vi "main 0.3.vi"() -> ()   [LabVIEW 2015]
uses:
  subvi/PHOIBOS/DEFINITIONS/DEF_dev_state.ctl
  subvi/PHOIBOS/DEFINITIONS/DEF_dev_type.ctl
  <vilib>/Utility/file.llb/Write Delimited Spreadsheet (I64).vi
  <vilib>/Utility/file.llb/Write Delimited Spreadsheet (DBL).vi
  subvi/Newport ESP301/Newport ESP301.lvlib
  subvi/sp_manip.llb/sp_manip_lib.lvlib
  subvi/sp_manip.llb/tcp_gateway.lvlib
panel:
  out "state":T1 items=["Off"=-1, "Standby"=0, "On"=1]
  in  "BasePath 2":path=path "Z:/PESdata"
  out "ESP_con?":bool caption="ESP301"
  out "phoib_con?":bool caption="PHOIBOS"
  out "manip_con?":bool caption="manipulator"
  out "cam_con?":bool caption="camera"
  in  "main_close":bool
  in  "Tab Control":enum32{"Live", "Measure", "Settings", "Devices"}(tab)
  out "cam_fps":dbl(slide)=8.239338102188393 caption="FPS" scale=0.1..50.0
  out "cam_burst_progress":u8(slide) scale=0.0..200.0
  in  "cam_burstnr":u32 max=1000
  in  "cam_burst":bool
  in  "ESP_delta":dbl
  in  "ESP_+ 2":bool
  in  "ESP_+":bool
  in  "ESP_go":bool
  in  "ESP_dest_t":dbl caption="Delay"
  in  "ESP_dest":dbl caption="Position"
  in  "ESP_set_t0":bool
  in  "phoib_I_6s":dbl=3200.0
  in  "phoib_I_5s":dbl=1400.0
  in  "phoib_I_4s":dbl=4.2
  in  "phoib_I_3s":dbl
  in  "phoib_I_2s":dbl=35.0
  in  "phoib_I_1s":dbl=21.9
  in  "phoib_standby":bool
  in  "phoib_set":bool
  out "phoib_I_6":dbl caption="Screen Voltage"
  out "phoib_I_5":dbl caption="Detctor Voltage"
  out "phoib_I_4":dbl caption="Work Function"
  out "phoib_I_3":dbl caption="Coil Current"
  out "phoib_I_2":dbl caption="Pass Energy"
  out "phoib_I_1":dbl caption="Kinetic Energy"
  out "CCD temp [°C]":i32=-12
  out "electronics temp [°C]":i32=30
  out "Saved Positions":string[][](table)=[["ertwertwert", "-2.299945", "-2.030214", "38.900024", "50.000762", "0.000887", "-97.998082"], ["uztgugt", "-14.999451", "-13.638894", "442.380066", "13.998380", "-1.893758", "-76.305838"], ["asdf", "-14.999451", "-13.638894", "442.380066", "13.998380", "-1.893758", "-76.305838"], ["test3", "-14.999451", "-13.638894", "441.380066", "13.998380", "-1.893758", "-76.305838"]]
  in  "Save Pos":bool
  in  "Load":bool
  in  "Delete":bool
  in  "ManipRel":dbl=1.0
  in  "ManipRel +":bool
  in  "ManipRel -":bool
  in  "manip.rel.select":enum32{"x", "y", "z", "polar", "tilt", "azimut"}(radio)=enum."polar"
  in  "Move Abs":bool
  in  "stop manip":bool
  in  "dest":dbl[](array[numeric])=[0.007141549166819264, -0.009888298846365134, 431.30615234375, 89.00040512814502, 1.109125024699864, -227.9162918846475] caption="destinations" format="%#.5g"
  out "names":string[](array[string])=["x", "y", "z", "polar", "tilt", "azimut"]
  out "pos":dbl[](array[numeric])=[0.007141549166819264, -0.009888298846365134, 431.30615234375, 89.00040512814502, 1.109125024699864, -227.9162918846475] caption="positions" format="%.5f"
  out "Intensity Graph":u16[][](graph)
  in  "Exposure [ms]":u32=20
  in  "Mode":T2(ring)=enum."WideAngleMode"
  in  "VoltageRange":enum16{"3.5kV", "1.5kV", "400V", "100V", "10V"}(ring)=enum."400V"
  out "ESP_pos":dbl caption="Position"
  out "ESP_delay":dbl caption="Delay"
  in  "ESP_t0":dbl caption="Time Zero @"
  in  "binning":u16(ring)=2 items=["X 1", "X 2", "X 4", "X 8"]
  in  "Gain":bool
  out "max value":u16=55
  out "phoib_I_7":dbl caption="Conversion Voltage"
  in  "phoib_I_7s":dbl
  in  "phoib_I_8s":dbl
  in  "phoib_I_9s":dbl
  out "phoib_I_8":dbl caption="FD1"
  out "phoib_I_9":dbl caption="FD2"
  out "opti_frames":dbl=25.0 caption="#steps_opti"
  out "opti_current_frame":i32=25
  out "Measurement Progress":u8(slide) scale=0.0..100.0
  out "Camera Aquisition":u8(slide) scale=0.0..100.0
  in  "Optimize":bool
  in  "OptiStepSize":dbl=-1.0 caption="Step Size"
  in  "OptiRange":dbl=25.0 caption="Range"
  in  "meas_axis":string(combo)="tilt" caption="Axis"
  in  "meas_avg":i32=60 caption="Frames2Average"
  in  "OptiCancel":bool
  out "#steps_opti":dbl=25.0
  out "current_step_opti":i32=25
  out "ETA":string
  in  "BasePath":path=path "Z:/PESdata"
  in  "Path":path=path "Z:/software/ManipulatorControl/save.txt"
  in  "ROI Bottom":i32=32
  in  "ROI Top":i32=1
  in  "ROI Right":i32=40
  in  "ROI Left":i32=1
  in  "ESP Axis":i32=1 min=1 max=3
  in  "manip_init":bool
  in  "manip_release":bool
  in  "phoib_init":bool
  in  "phoib_release":bool
  in  "ESP_init":bool
  in  "ESP_release":bool
  in  "ESP301 VISA":refnum<visa-resource-name>="COM8"
  in  "cam_boardnr":i32
  in  "cam_init":bool
  in  "cam_release":bool
  out "error out":errorcluster
  out "error out 2":errorcluster
  # "step _ of _"
  # "step _ of _"
  # "manip"
  # "phoib"
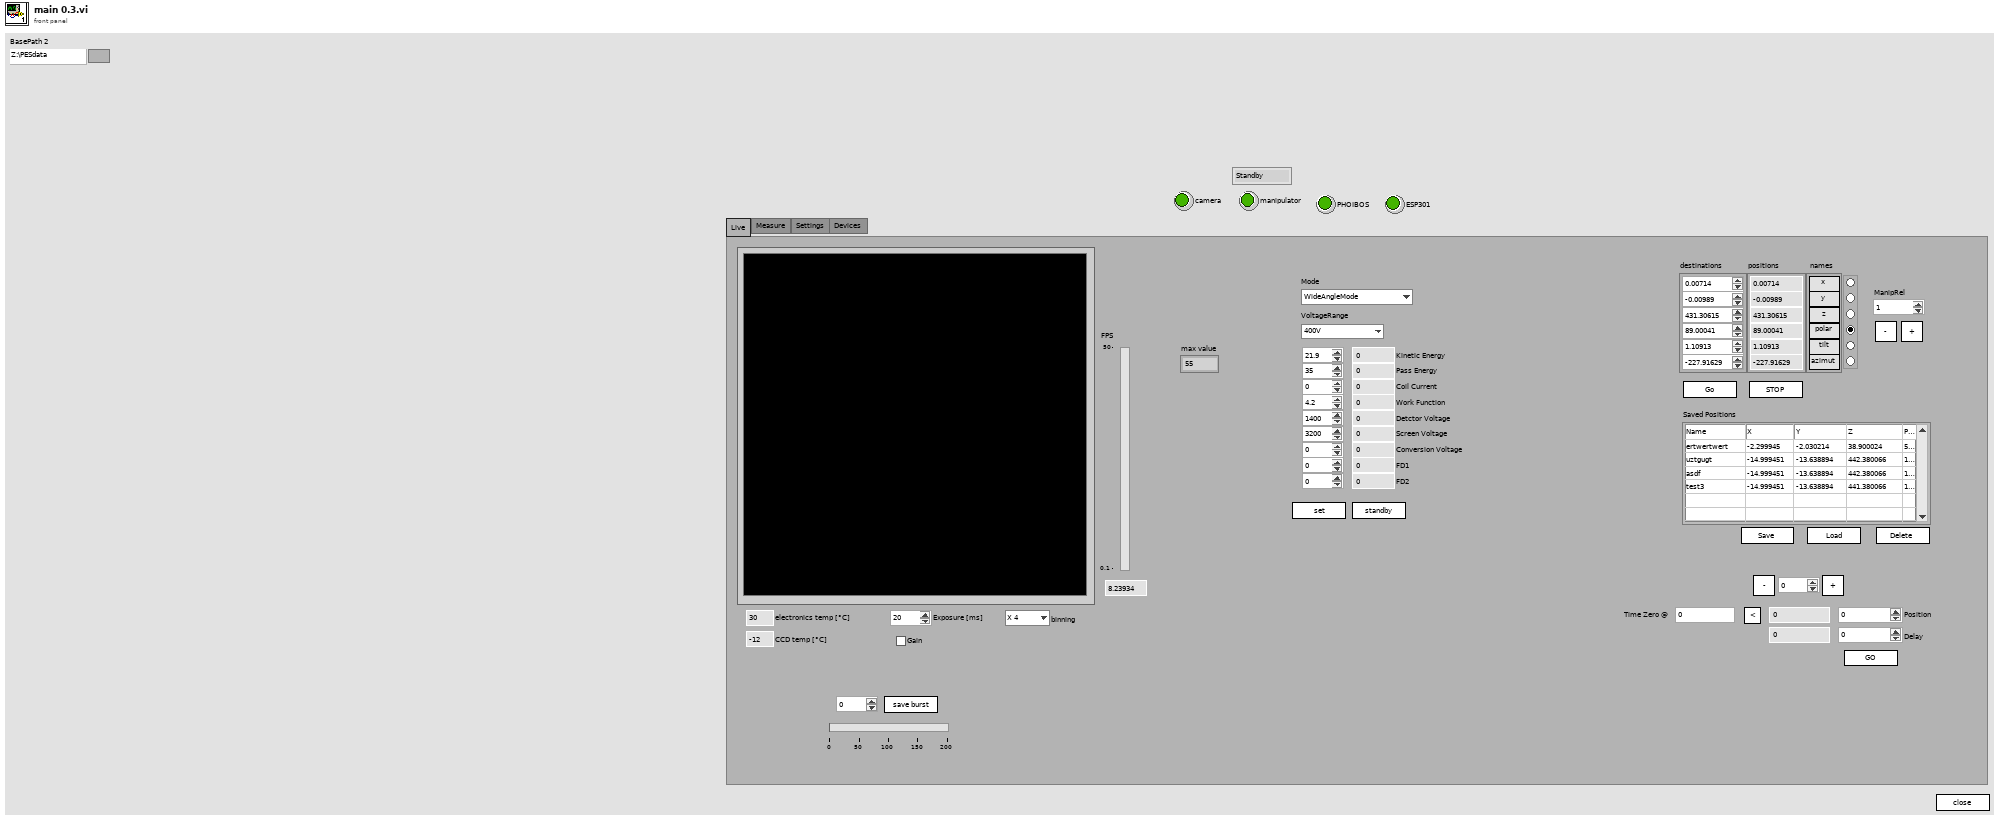
[diagram p1: front panel]
types:
  T1 = typedef "DEF_dev_state.ctl" = i32
  T2 = enum16{"HighMagnification", "MediumMagnification", "LowMagnification", "HighAngularDispersion", "MediumAngularDispersion", "LowAngularDispersion", "WideAngleMode", "LargeArea", "MediumArea", "SmallArea", "HighMagnification2", "SmallArea2", "ImagingMode"}
  T3 = cluster{"Camera type":u32, "Operating mode\nHP & QE / HS & DiCam Pro ":u32, "Frame trigger \n(High Performance and QE only)":u16, "Sequence trigger":u16, "Low Light\n(QE only)":bool, "Gain":bool, "Horzontal\nbinning":u16, "Vertical\nbinning ":u16, "ROI Left":i32, "ROI Right":i32, "ROI Top":i32, "ROI Bottom":i32}
  T4 = enum16{"open", "replace", "create", "open or create", "replace or create", "replace or create with confirmation"}
  T5 = cluster{"Axis_Name":string, "Axis_Type":string, "Axis_Position":dbl, "continous":bool, "moving":bool}[]
  T6 = cluster{"Axis_Name":string, "Axis_Type":string, "Axis_Position":dbl, "continous":bool, "moving":bool}
  T7 = typedef "DEF_dev_type.ctl" = enum32{"devA (analyzer)", "devD (detector)"}
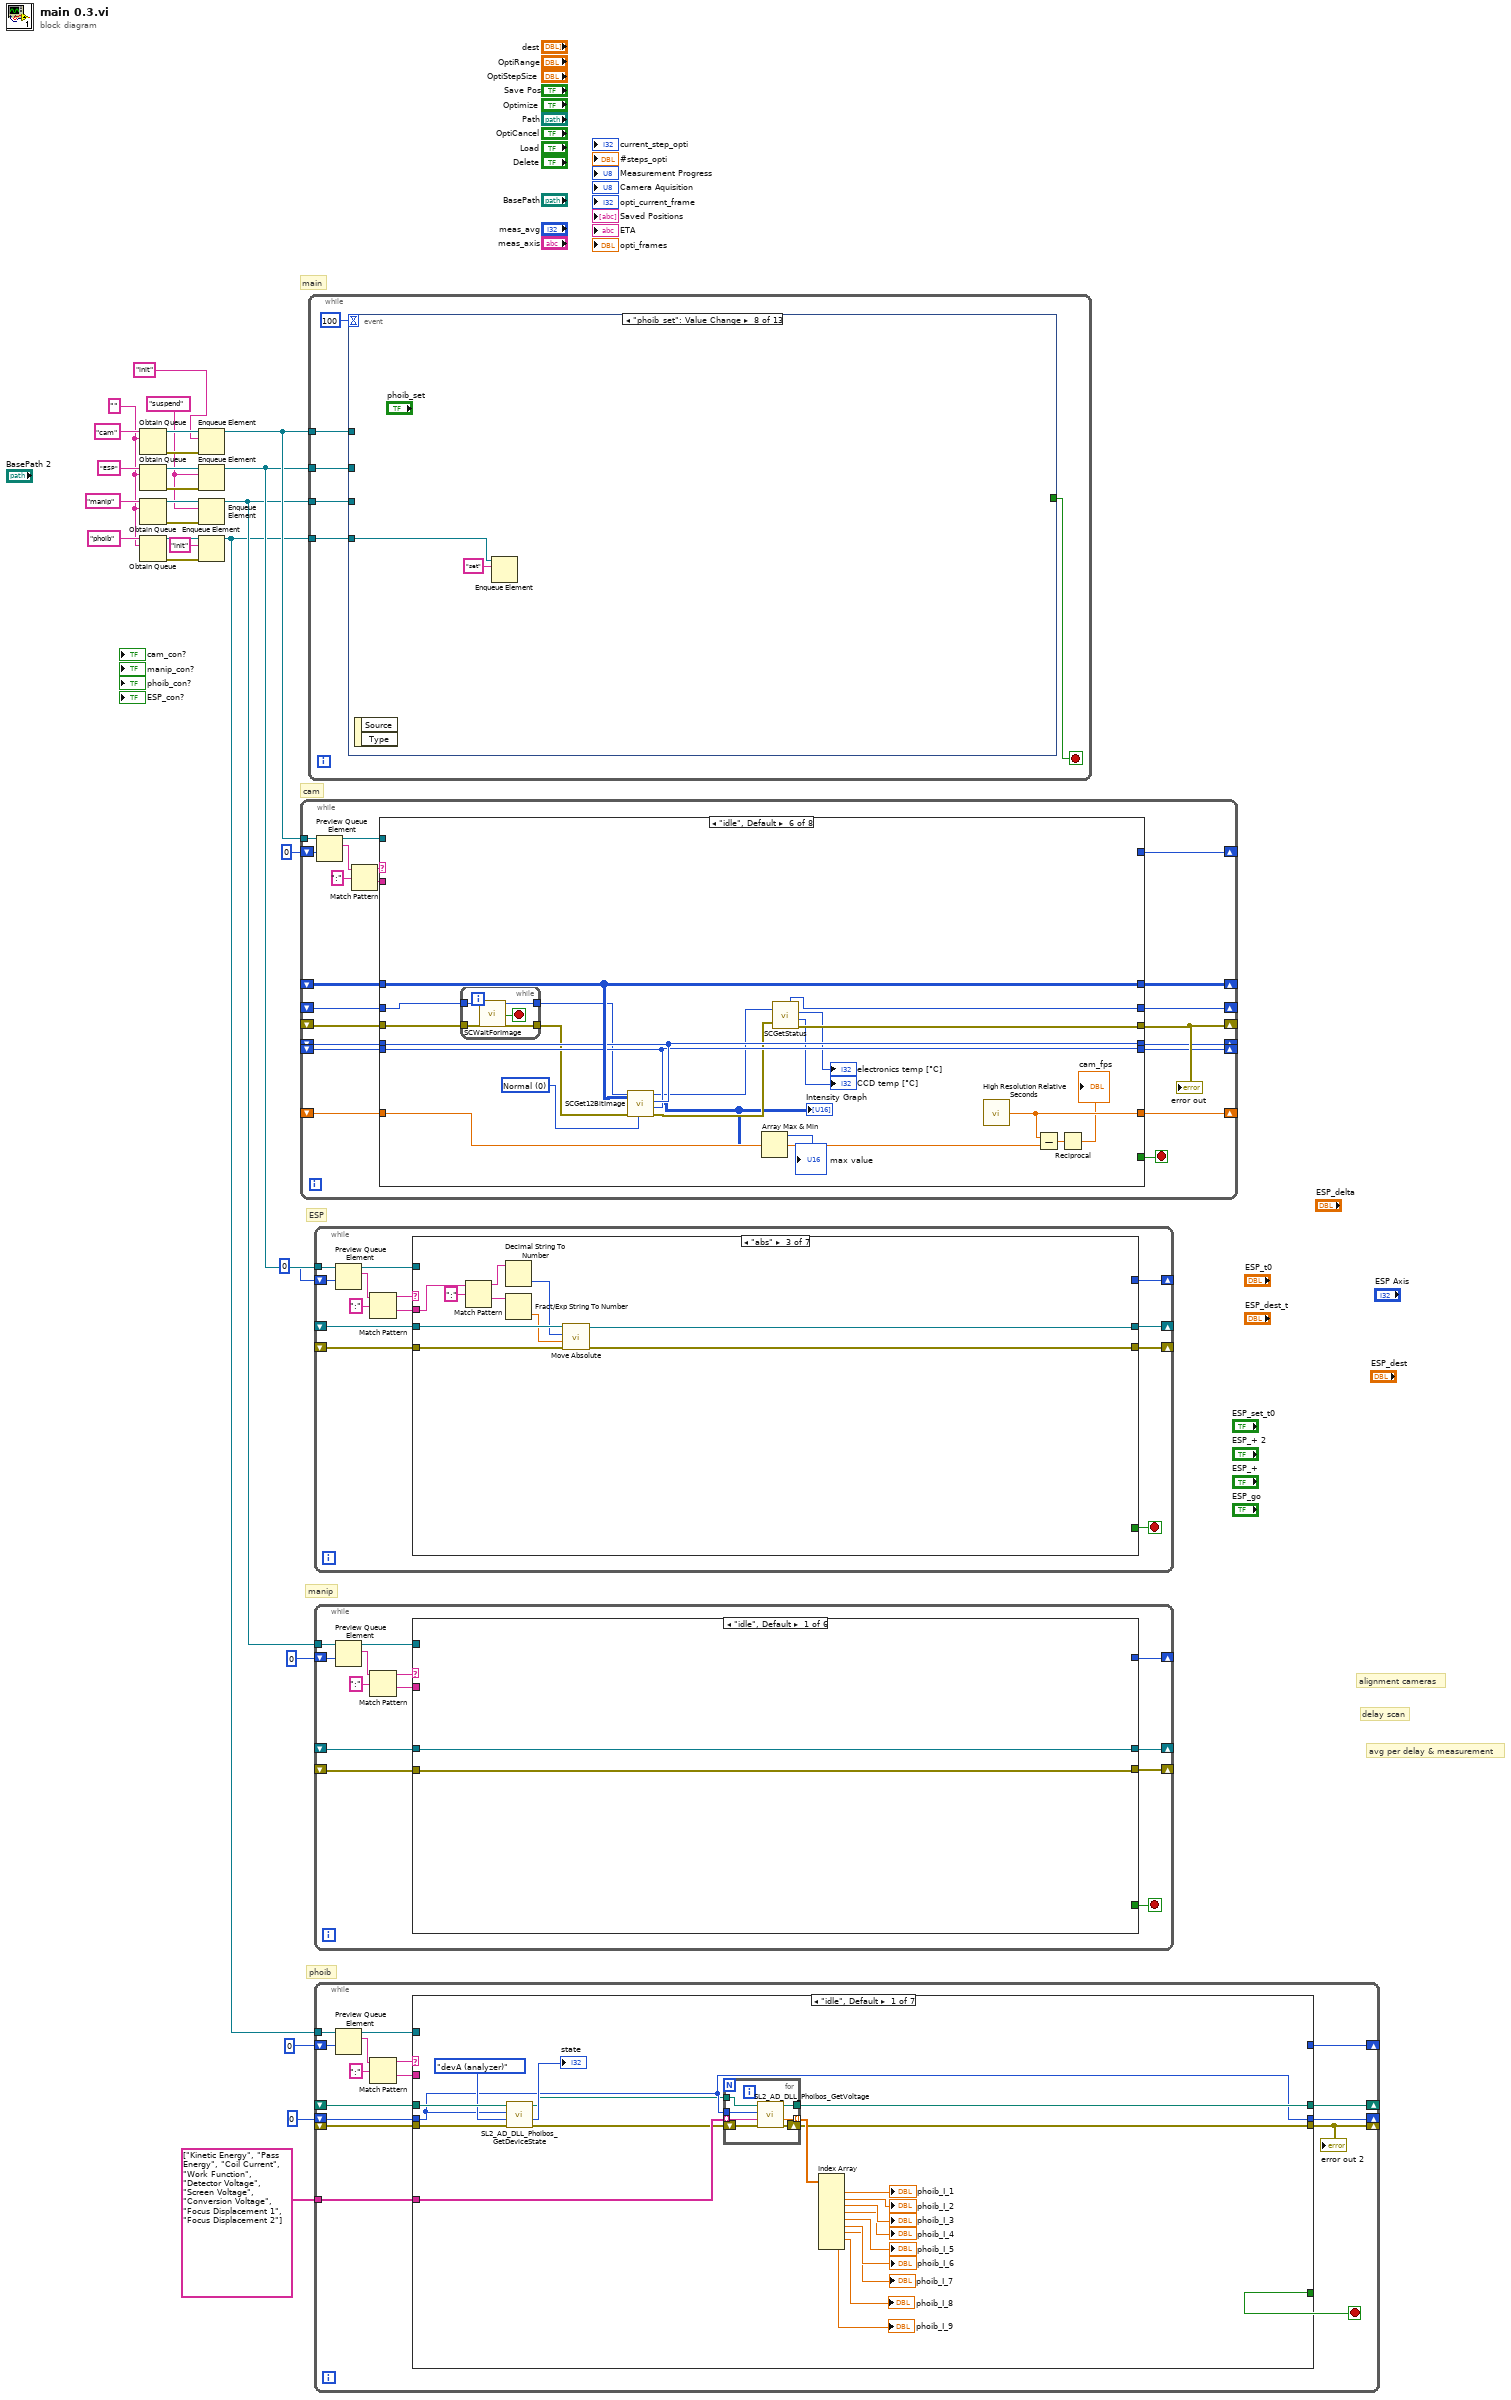
[diagram p0: block diagram]
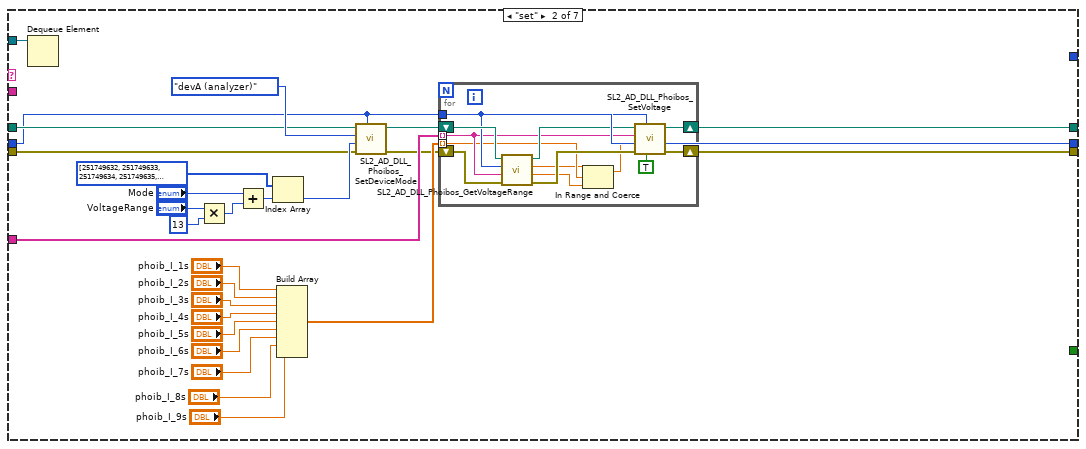
[diagram p2: hidden frame]
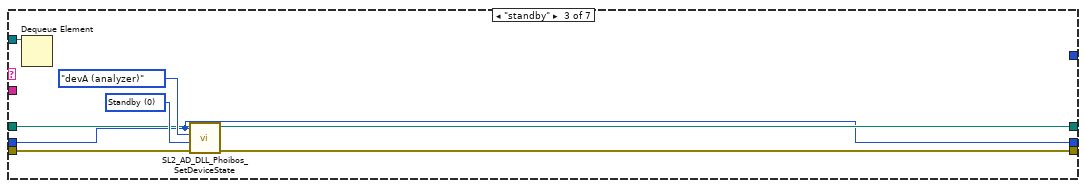
[diagram p3: hidden frame]
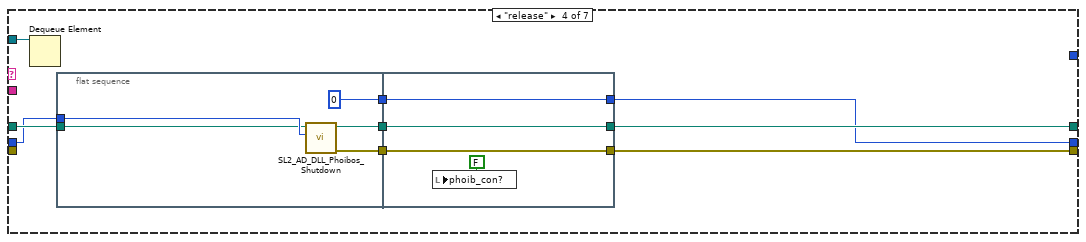
[diagram p4: hidden frame]
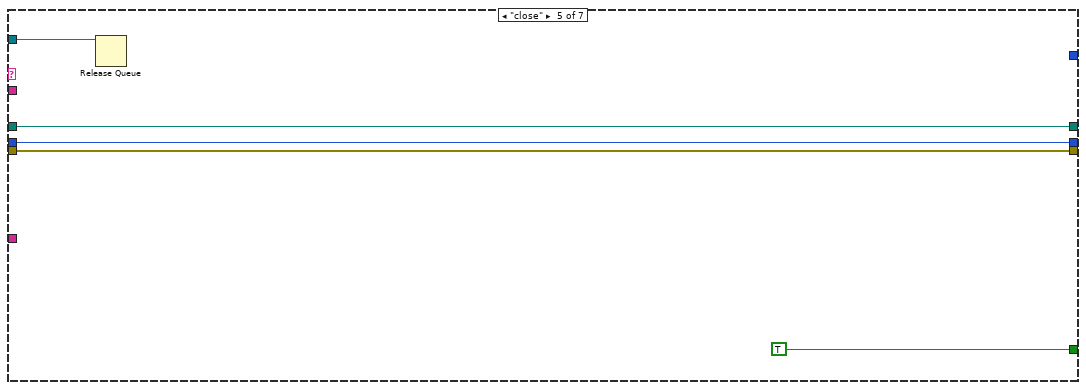
[diagram p5: hidden frame]
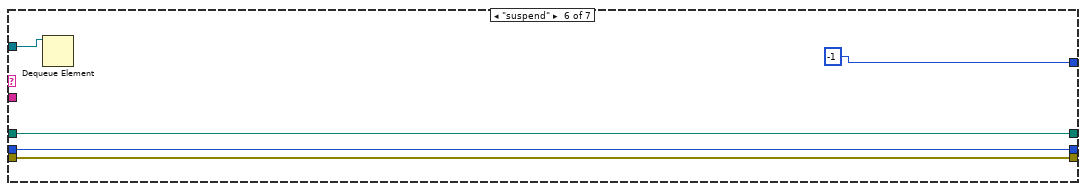
[diagram p6: hidden frame]
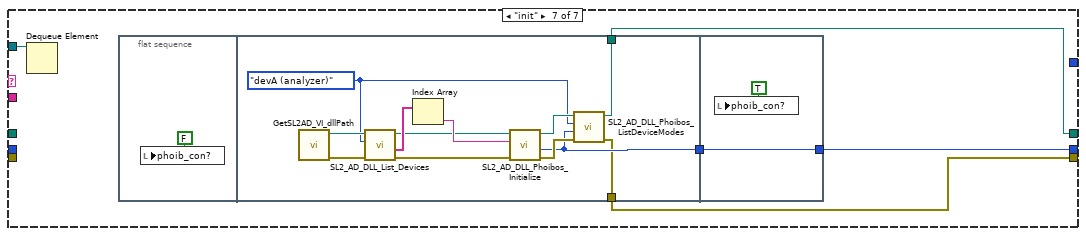
[diagram p7: hidden frame]
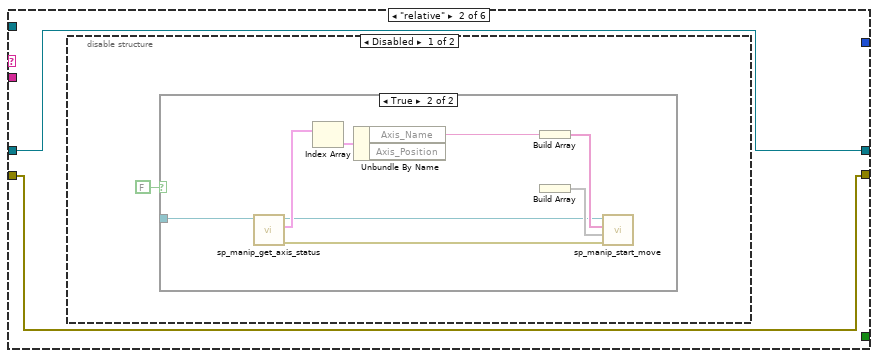
[diagram p8: hidden frame]
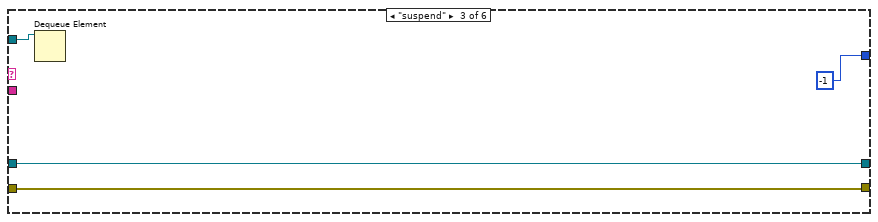
[diagram p11: hidden frame]
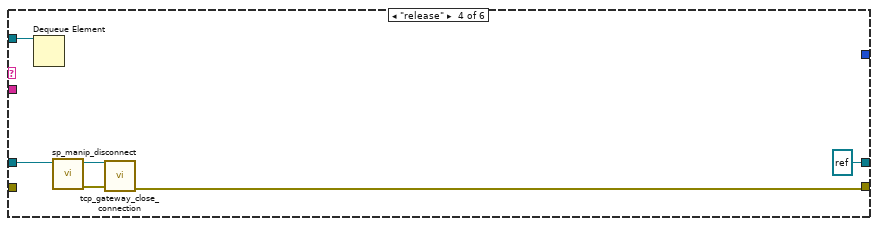
[diagram p12: hidden frame]
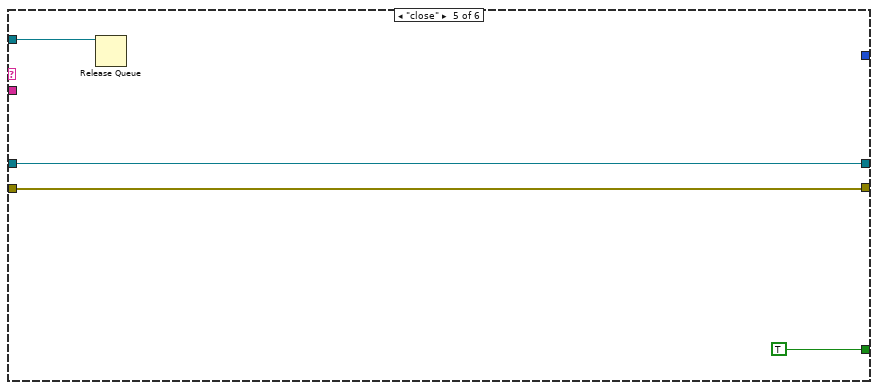
[diagram p13: hidden frame]
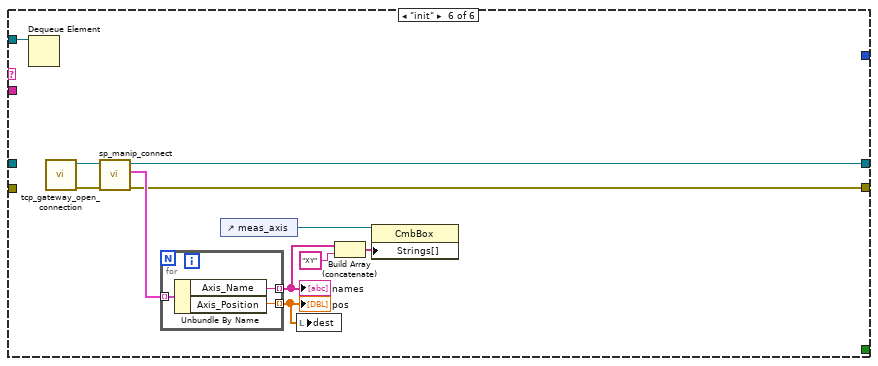
[diagram p14: hidden frame]
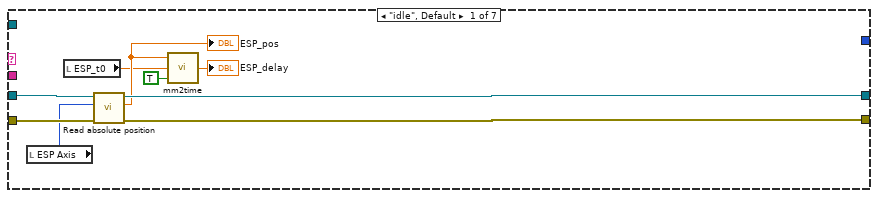
[diagram p15: hidden frame]
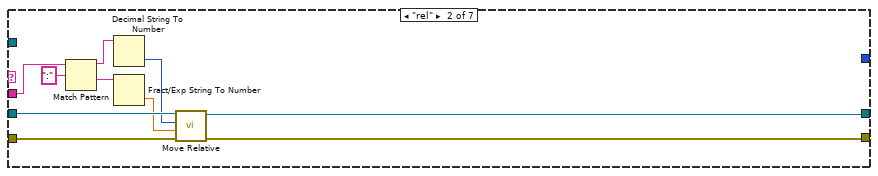
[diagram p16: hidden frame]
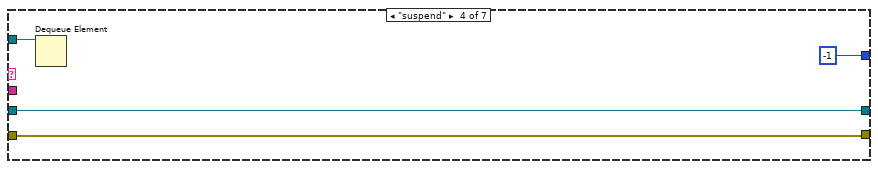
[diagram p17: hidden frame]
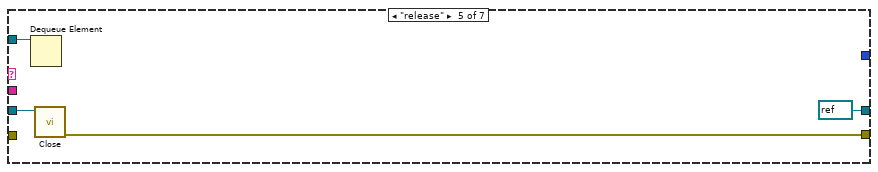
[diagram p18: hidden frame]
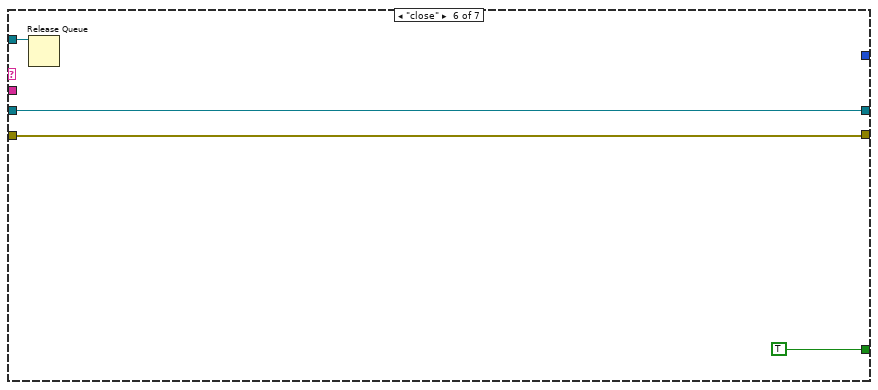
[diagram p19: hidden frame]
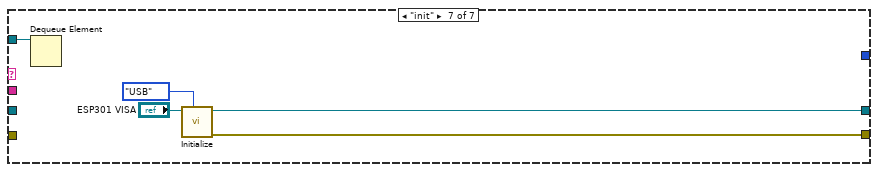
[diagram p20: hidden frame]
diagram:
  w13 = "suspend" ("name (unnamed)")
  w12 = "" ("name (unnamed)")
  # "avg per delay & measurement"
  # "delay scan"
  # "alignment cameras"
  # "phoib"
  # "manip"
  # "ESP"
  # "cam"
  # "main"
  n1 = Obtain Queue(name (unnamed)="cam", element data type=w12) -> (queue out=w25:refnum<queue>, error out=w24:errorcluster)  [unwired: 3 in, 1 out]
  n2 = Obtain Queue(name (unnamed)="ESP", element data type=w12) -> (queue out=w21:refnum<queue>, error out=w22:errorcluster)  [unwired: 3 in, 1 out]
  n3 = Obtain Queue(name (unnamed)="manip", element data type=w12) -> (queue out=w18:refnum<queue>, error out=w17:errorcluster)  [unwired: 3 in, 1 out]
  n4 = Obtain Queue(name (unnamed)="phoib", element data type=w12) -> (queue out=w15:refnum<queue>, error out=w16:errorcluster)  [unwired: 3 in, 1 out]
  n5 = Enqueue Element(queue=w25, element="init" ("name (unnamed)"), error in (no error)=w24) -> (queue out=w23:refnum<queue>)  [unwired: 1 in, 2 out]
  n6 = Enqueue Element(queue=w21, element=w13, error in (no error)=w22) -> (queue out=w11:refnum<queue>)  [unwired: 1 in, 2 out]
  n7 = Enqueue Element(queue=w18, element=w13, error in (no error)=w17) -> (queue out=w10:refnum<queue>)  [unwired: 1 in, 2 out]
  n8 = Enqueue Element(queue=w15, element="init", error in (no error)=w16) -> (queue out=w9:refnum<queue>)  [unwired: 1 in, 2 out]
  n9 = while {
    tunnel: w23 -> [w47]
    shift-right: [w41] -> _
    shift-left: _ -> [w40]
    shift-right: [w39] -> _
    shift-left: _ -> [w35]
    shift-right: [w38] -> _
    shift-left: _ -> [w34]
    shift-right: [w37] -> _
    shift-left: _ -> [w33]
    shift-right: [w36] -> _
    shift-left: _ -> [w32]
    shift-right: [w29] -> _
    shift-left: 0 -> [w30]
    shift-right: [w28] -> _
    shift-left: _ -> [w27]
    stop <- w31 stop-if-true
    n10 = Preview Queue Element(queue=w47, timeout in ms (-1)=w30) -> (queue out=w46:refnum<queue>, element=w45:string)  [unwired: 1 in, 2 out]
    n11 = Match Pattern(string=w45, regular expression=":") -> (before substring=w42:string, after substring=w43:string)  [unwired: 1 in, 2 out]
    n12 = case shown="\"idle\", Default" w42 {
      tunnel: w46 -> [w56 w80 w123 w168 w179 _ _ w235]
      tunnel: w43 -> [_ _ w136 _ _ _ w211 _]
      tunnel: [u16[][] [] w81 w133 w167 w177 w199 w209 w233] -> w41
      tunnel: w40 -> [_ _ w133 w167 w177 w199 w209 w233]
      tunnel: [w55 w82 w132 u64 0 ("Hout") w176 w190 w208 w232] -> w39
      tunnel: [w57 w83 w129 w162 w175 w193 w207 w231] -> w38
      tunnel: [0 ("Horizontal size") w73 w131 w166 w174 w198 w206 w230] -> w37
      tunnel: [0 ("Vertical size") w72 w130 w165 w173 w197 w205 w229] -> w36
      tunnel: w35 -> [_ w85 w132 w164 w176 w189 w208 w232]
      tunnel: w34 -> [_ w84 w129 _ w175 w188 w218 w231]
      tunnel: w33 -> [_ _ w131 w166 w174 w198 w206 w230]
      tunnel: w32 -> [_ _ w130 w165 w173 w197 w205 w229]
      tunnel: [_ _ _ _ TRUE _ _ _] -> w31
      tunnel: [_ _ _ _ _ _ _ -1] -> w29
      tunnel: [_ _ _ _ _ w185 _ _] -> w28
      tunnel: w27 -> [_ _ _ _ _ w184 _ _]
      frame "init" {
        n13 = Dequeue Element(queue=w56) -> (queue out=w49:refnum<queue>)  [unwired: 2 in, 3 out]
        n14 = Enqueue Element At Opposite End(queue=w49, element="set") -> ()  [unwired: 2 in, 3 out]
        n15 = flat-sequence {
          tunnel: [w59] -> w54
          tunnel: [w60] -> w53
          tunnel: [w68] -> w55
          tunnel: [w69] -> w57
          tunnel: w54 -> [w69]
          tunnel: w53 -> [w68]
          frame #0 {
            n16 = local write "cam_con?"(FALSE ("cam_con?")) -> ()
          }
          frame #1 {
            n17 = call "SCInitBoard.vi"("boardnr"="cam_boardnr") -> ("Hout"=w63:u32, "error out"=w64:errorcluster)  [unwired: 1 in, 1 out]
            n18 = call "SCSetupCamera.vi"("Handle"=w63, "error in (no error)"=w64) -> ("Hout"=w65:u64, "error out"=w66:errorcluster)  [unwired: 1 out]
            n19 = call "SCStopCOC.vi"("error in (no error)"=w66, "Stop mode"=0, "Handle"=w65) -> ("error out"=w59:errorcluster, "Hout"=w60:u64)
          }
          frame #2 {
            n20 = local write "cam_con?"(TRUE ("cam_con?")) -> ()
          }
        }
      }
      frame "set" {
        w79 = u32 1 ("Operating mode\nHP & QE / HS & DiCam Pro")
        n21 = Dequeue Element(queue=w80) -> ()  [unwired: 2 in, 4 out]
        n22 = Bundle By Name(cluster=cluster{"Delay":dbl, "Exposure ":dbl} {"Delay"=0.0, "Exposure "=0.0} ("Delay and exposure"), "Exposure"="Exposure [ms]") -> (w76:cluster{"Delay":dbl, "Exposure ":dbl})
        n23 = Bundle By Name(cluster=T3 {"Camera type"=0, "Operating mode\nHP & QE / HS & DiCam Pro "=0, "Frame trigger \n(High Performance and QE only)"=0, "Sequence trigger"=0, "Low Light\n(QE only)"=FALSE, "Gain"=FALSE, "Horzontal\nbinning"=0, "Vertical\nbinning "=0, "ROI Left"=1, "ROI Right"=20, "ROI Top"=1, "ROI Bottom"=15} ("Camera controls"), "Operating mode\nHP & QE / HS & DiCam Pro"=w79, "Horzontal\nbinning"="binning", "Vertical\nbinning"="binning", "ROI Left"="ROI Left", "ROI Right"="ROI Right", "ROI Top"="ROI Top", "ROI Bottom"="ROI Bottom", "Gain"="Gain") -> (w96:T3)
        n24 = call "New delay and exposure forma.vi"("Operating mode\nHP & QE / HS & DiCam Pro"=w79, "Delay and exposure"=w76) -> ("Output table"=w97:string)  [unwired: 3 in]
        n25 = call "SCStopCOC.vi"("error in (no error)"=w84, "Stop mode"=0, "Handle"=w85) -> ("error out"=w101:errorcluster, "Hout"=w100:u64)
        n26 = call "SCSetCoC.vi"("error in (no error)"=w101, "Delay and exposure table"=w97, "Camera controls"=w96, "Handle"=w100) -> ("error out"=w89:errorcluster, "Hout"=w88:u64)  [unwired: 1 out]
        n27 = call "SCGetImageSize.vi"("Handle"=w88, "error in (no error)"=w89) -> ("Hout"=w87:u64, "error out"=w86:errorcluster, "Horizontal size"=w73:i32, "Vertical size"=w72:i32)  [unwired: 2 out]
        n28 = Greater?(x=w73, y=w72) -> (0:w74:bool)
        n29 = Select(t=w73, s=w74, f=w72) -> (s? t:f=w71:i32)
        n30 = Initialize Array(u16 0 ("dimension size"), w72, w73) -> (w81:u16[][])
        n31 = call "SCRun.vi"("error in (no error)"=w86, "Run mode"=0, "Handle"=w87) -> ("error out"=w83:errorcluster, "Hout"=w82:u64)  [unwired: 1 out]
        n32 = property on="Intensity Graph" class="IntGraph (strict)"("XScale.Maximum"=w71, "YScale.Maximum"=w71) -> ()  [unwired: 2 in, 2 out]
      }
      frame "burst" {
        w103 = "\r"
        w104 = "\t"
        n33 = local read "Exposure [ms]"() -> (w112:u32)
        n34 = local read "binning"() -> (w114:u16)
        n35 = Dequeue Element(queue=w123) -> ()  [unwired: 2 in, 4 out]
        n36 = local read "Gain"() -> (w113:bool)
        n37 = Boolean To (0,1)(Boolean=w113) -> (0, 1=w115:i16)
        n38 = Get Date/Time In Seconds() -> (seconds since 1Jan1904=w128:timestamp)
        n39 = Match Pattern(string=w136, regular expression=":") -> (before substring=w135:string, after substring=w134:string)  [unwired: 1 in, 2 out]
        n40 = Number To Decimal String(number=w112) -> (decimal integer string=w117:string)  [unwired: 1 in]
        n41 = Number To Decimal String(number=w115) -> (decimal integer string=w119:string)  [unwired: 1 in]
        n42 = Number To Decimal String(number=w114) -> (decimal integer string=w121:string)  [unwired: 1 in]
        n43 = String To Path(string=w134) -> (path=w126:path)
        n44 = Format Date/Time String(time format string (%c)="%Y.%m.%d-%H.%M.%S", seconds (now)=w128) -> (date/time string=w125:string)  [unwired: 1 in]
        n45 = Build Path(base path=w126, name or relative path=w125) -> (appended path=w124:path)
        n46 = Decimal String To Number(string=w135) -> (number=w102:i32)  [unwired: 2 in, 1 out]
        n47 = Create Folder(path (use dialog)=w124) -> (created path=w107:path)  [unwired: 2 in, 2 out]
        n48 = Concatenate Strings("Exposure:", w104, w117, w103, "Gain:", w104, w119, w103, "binning", w104, w121, w103) -> (w111:string)
        n49 = Build Path(base path=w107, name or relative path="info.txt") -> (appended path=w106:path)
        n50 = Open/Create/Replace File(file path (use dialog)=w106, operation (0:open)=T4."replace or create") -> (refnum out=w109:refnum<file>)  [unwired: 4 in, 2 out]
        n51 = Write to Text File(file (use dialog)=w109, text=w111) -> (refnum out=w110:refnum<file>)  [unwired: 2 in, 2 out]
        n52 = Close File(refnum=w110) -> ()  [unwired: 1 in, 2 out]
        n53 = for {
          N: w102 -> [_]
          tunnel: w133 -> [w154]
          tunnel: w132 -> [w151]
          tunnel: w129 -> [w150]
          tunnel: w131 -> [w153]
          tunnel: w130 -> [w152]
          tunnel: w107 -> [w145]
          tunnel: 1000 ("x") -> [w143]
          i -> [w138]
          w155 = 0 items=["Normal", "Upside down"] ("mode")
          n54 = while {
            tunnel: [w159] -> w148
            tunnel: [w158] -> w149
            tunnel: w151 -> [w157]
            tunnel: w150 -> [w156]
            stop <- w160 stop-if-true
            n55 = call "SCWaitForImage.vi"("Handle"=w157, "error in (no error)"=w156) -> ("Hout"=w158:u64, "Image Valid"=w160:bool, "error out"=w159:errorcluster)  [unwired: 15 in]
          }
          n56 = Add(x=w143, y=w138) -> (x+y=w142:i32)
          n57 = Number To Decimal String(number=w142) -> (decimal integer string=w141:string)  [unwired: 1 in]
          n58 = String Subset(string=w141, offset (0)=1) -> (substring=w139:string)  [unwired: 1 in]
          n59 = Build Path(base path=w145, name or relative path=w139) -> (appended path=w144:path)
          n60 = call "SCGet12BitImage.vi"("mode"=w155, "Input array"=w154, "error in (no error)"=w148, "Vertical size"=w152, "Horizontal size"=w153, "Handle"=w149) -> ("error out"=w146:errorcluster, "imgdata"=w147:u16[][])  [unwired: 1 in, 1 out]
          n61 = call-poly <vilib>:"Write Delimited Spreadsheet.vi"("file path (dialog if empty)"=w144, "2D data"=w147, "error in (no error)"=w146) -> ()  [unwired: 11 in, 2 out]
          n62 = local write "Intensity Graph"(w147) -> ()
          "cam_burst_progress" <- w138
        }
        n63 = property on="cam_burst_progress" class="Slide (strict)"("Scale.Maximum"=w102) -> ()  [unwired: 2 in, 2 out]
      }
      frame "release" {
        n64 = Dequeue Element(queue=w168) -> ()  [unwired: 2 in, 4 out]
        n65 = flat-sequence {
          tunnel: w164 -> [w170]
          tunnel: [w169] -> w161
          tunnel: [w172] -> w162
          tunnel: w161 -> [w172]
          frame #0 {
            n66 = call "SCCloseBoard.vi"("Handle"=w170) -> ("error out"=w169:errorcluster)  [unwired: 1 in, 2 out]
          }
          frame #1 {
            n67 = local write "cam_con?"(FALSE ("cam_con?")) -> ()
          }
        }
      }
      frame "close" {
        n68 = Release Queue(queue=w179) -> ()  [unwired: 2 in, 3 out]
      }
      frame "idle", Default {
        w196 = 0 items=["Normal", "Upside down"] ("mode")
        n69 = while {
          tunnel: [w203] -> w186
          tunnel: [w202] -> w187
          tunnel: w189 -> [w201]
          tunnel: w188 -> [w200]
          stop <- w204 stop-if-true
          n70 = call "SCWaitForImage.vi"("Handle"=w201, "error in (no error)"=w200) -> ("Hout"=w202:u64, "Image Valid"=w204:bool, "error out"=w203:errorcluster)  [unwired: 15 in]
        }
        n71 = call "SCGet12BitImage.vi"("mode"=w196, "Input array"=w199, "error in (no error)"=w186, "Vertical size"=w197, "Horizontal size"=w198, "Handle"=w187) -> ("error out"=w194:errorcluster, "imgdata"=w181:u16[][], "Hout"=w195:u64)  [unwired: 1 in]
        "Intensity Graph" <- w181
        n72 = Array Max & Min(array=w181) -> (max value=→"max value":u16)  [unwired: 3 out]
        n73 = call "SCGetStatus.vi"("Handle"=w195, "error in (no error)"=w194) -> ("Hout"=w190:u64, "Electronics temperature"=→"electronics temp [°C]":i32, "CCD temperature"=→"CCD temp [°C]":i32, "error out"=w193:errorcluster)  [unwired: 2 out]
        n74 = call <vilib>:"High Resolution Relative Seconds.vi"() -> ("relative seconds"=w185:dbl)
        n75 = Subtract(x=w185, y=w184) -> (x-y=w183:dbl)
        n76 = Reciprocal(x=w183) -> (1/x=→"cam_fps":dbl)
      }
      frame "snap" {
        n77 = local read "BasePath 2"() -> (w220:path)
        n78 = local read "meas_avg"() -> (w215:i32)
        n79 = Initialize Array(u32 0 ("element"), w206, w205) -> (w217:u32[][])
        n80 = Build Path(base path=w220, name or relative path=w211) -> (appended path=w210:path)
        n81 = for {
          N: w215 -> [_]
          tunnel: w206 -> [w228]
          tunnel: w205 -> [w227]
          tunnel: w209 -> [w225]
          shift-right: [w222] -> w216
          shift-left: w217 -> [w224]
          shift-right: [w221] -> w207
          shift-left: w218 -> [w226]
          n82 = call "SCGet12BitImage.vi"("Input array"=w225, "error in (no error)"=w226, "Vertical size"=w227, "Horizontal size"=w228) -> ("error out"=w221:errorcluster, "imgdata"=w223:u16[][])  [unwired: 3 in, 1 out]
          n83 = Add(x=w223, y=w224) -> (x+y=w222:u32[][])
        }
        n84 = Divide(x=w216, y=w215) -> (x/y=w214:dbl[][])
        n85 = call-poly <vilib>:"Write Delimited Spreadsheet.vi"("file path (dialog if empty)"=w210, "format (%.3f)"="%d", "2D data"=w214, "transpose? (F)"=TRUE) -> ()  [unwired: 10 in, 2 out]
      }
      frame "suspend" {
        n86 = Dequeue Element(queue=w235) -> ()  [unwired: 2 in, 4 out]
      }
    }
    "error out" <- w38
  }
  n87 = while {
    tunnel: w23 -> [w239]
    tunnel: w11 -> [w238]
    tunnel: w10 -> [w237]
    tunnel: w9 -> [w236]
    stop <- w241 stop-if-true
    n88 = event shown="[7] \"phoib_set\": Value Change" {
      selector: _ -> [_ _ _ _ _ _ _ _ _ _ _ _ _]
      dyn-events: _ -> [_ _ _ _ _ _ _ _ _ _ _ _ _]
      timeout: 100 -> [_ _ _ _ _ _ _ _ _ _ _ _ _]
      tunnel: [_ TRUE _ _ _ _ _ _ _ _ _ _ _] -> w241
      tunnel: w239 -> [_ w251 w254 _ _ _ _ _ w280 w281 _ _ _]
      tunnel: w238 -> [_ w250 _ w258 _ _ _ _ _ _ _ _ _]
      tunnel: w237 -> [_ w249 _ _ w264 _ _ _ _ _ _ _ _]
      tunnel: w236 -> [_ w248 _ _ _ w270 w276 w277 _ _ _ _ _]
      event Timeout {
        n89 = event-data() -> ()  [unwired: 1 in, 1 out]
      }
      event "main_close": Value Change {
        w242 = "close" ("element")
        w247 = "release" ("element")
        n90 = event-data() -> ()  [unwired: 1 in, 1 out]
        n91 = Enqueue Element(queue=w251, element=w247) -> (queue out=w246:refnum<queue>)  [unwired: 2 in, 2 out]
        n92 = Enqueue Element(queue=w250, element=w247) -> (queue out=w245:refnum<queue>)  [unwired: 2 in, 2 out]
        n93 = Enqueue Element(queue=w249, element=w247) -> (queue out=w244:refnum<queue>)  [unwired: 2 in, 2 out]
        n94 = Enqueue Element(queue=w248, element=w247) -> (queue out=w243:refnum<queue>)  [unwired: 2 in, 2 out]
        n95 = Enqueue Element(queue=w246, element=w242) -> ()  [unwired: 2 in, 3 out]
        n96 = Enqueue Element(queue=w245, element=w242) -> ()  [unwired: 2 in, 3 out]
        n97 = Enqueue Element(queue=w244, element=w242) -> ()  [unwired: 2 in, 3 out]
        n98 = Enqueue Element(queue=w243, element=w242) -> ()  [unwired: 2 in, 3 out]
      }
      event "cam_release", "cam_init": Value Change {
        n99 = event-data() -> ()  [unwired: 1 in, 2 out]
        n100 = Select(t="init" ("name (unnamed)"), s="cam_init", f="release" ("name (unnamed)")) -> (s? t:f=w253:string)
        n101 = Enqueue Element(queue=w254, element=w253) -> ()  [unwired: 2 in, 3 out]
      }
      event "ESP_release", "ESP_init": Value Change {
        n102 = event-data() -> ()  [unwired: 1 in, 2 out]
        n103 = Select(t="init" ("name (unnamed)"), s="ESP_init", f="release" ("name (unnamed)")) -> (s? t:f=w262:string)
        n104 = Enqueue Element(queue=w258, element=w262) -> ()  [unwired: 2 in, 3 out]
      }
      event "manip_init", "manip_release": Value Change {
        n105 = event-data() -> ()  [unwired: 1 in, 2 out]
        n106 = Flush Queue(queue=w264) -> (queue out=w263:refnum<queue>)  [unwired: 1 in, 2 out]
        n107 = Select(t="init" ("name (unnamed)"), s="manip_init", f="release" ("name (unnamed)")) -> (s? t:f=w266:string)
        n108 = Enqueue Element(queue=w263, element=w266) -> ()  [unwired: 2 in, 3 out]
      }
      event "phoib_release", "phoib_init": Value Change {
        n109 = event-data() -> ()  [unwired: 1 in, 2 out]
        n110 = Flush Queue(queue=w270) -> (queue out=w269:refnum<queue>)  [unwired: 1 in, 2 out]
        n111 = Select(t="init" ("name (unnamed)"), s="phoib_init", f="release" ("name (unnamed)")) -> (s? t:f=w272:string)
        n112 = Enqueue Element(queue=w269, element=w272) -> ()  [unwired: 2 in, 3 out]
      }
      event "phoib_standby": Value Change {
        n113 = event-data() -> ()  [unwired: 1 in, 2 out]
        n114 = Enqueue Element(queue=w276, element="standby") -> ()  [unwired: 2 in, 3 out]
      }
      event "phoib_set": Value Change {
        n115 = event-data() -> ()  [unwired: 1 in, 2 out]
        n116 = Enqueue Element(queue=w277, element="set") -> ()  [unwired: 2 in, 3 out]
      }
      event "ROI Left", "ROI Right", "ROI Top", "ROI Bottom", "Exposure [ms]", "binning", "Gain": Value Change {
        n117 = event-data() -> ()  [unwired: 1 in, 6 out]
        n118 = Enqueue Element(queue=w280, element="set") -> ()  [unwired: 2 in, 3 out]
      }
      event "cam_burst": Value Change {
        n119 = event-data() -> ()  [unwired: 1 in, 1 out]
        n120 = local read "BasePath"() -> (w285:path)
        n121 = call "File Dialog"("start path"=w285) -> ("selected path"=w283:path, "cancelled"=w284:bool, "error out"=w282:errorcluster)  [unwired: 11 in, 1 out]
        n122 = case shown="False" w284 {
          tunnel: w283 -> [w288 _]
          tunnel: w282 -> [_ _]
          tunnel: w281 -> [w293 _]
          frame False {
            n123 = Path To String(path=w288) -> (string=w287:string)
            n124 = Number To Decimal String(number="cam_burstnr") -> (decimal integer string=w290:string)  [unwired: 1 in]
            n125 = Concatenate Strings("burst:" ("string"), w290, ":" ("string"), w287) -> (w286:string)
            n126 = Enqueue Element(queue=w293, element=w286) -> ()  [unwired: 2 in, 3 out]
          }
          frame True {
          }
        }
      }
      event "Move Abs": Value Change {
        n127 = event-data() -> ()  [unwired: 1 in, 1 out]
      }
      event "ManipRel +", "ManipRel -": Value Change {
        n128 = event-data() -> ()  [unwired: 1 in, 2 out]
        n129 = Negate(x="ManipRel") -> (-x=w295:dbl)
        n130 = Select(t=w295, s="ManipRel -", f="ManipRel") -> ()  [unwired: 1 out]
      }
      event "stop manip": Value Change {
        n131 = event-data() -> ()  [unwired: 1 in, 1 out]
      }
    }
  }
  n132 = while {
    tunnel: w11 -> [w304]
    shift-right: [w302] -> _
    shift-left: _ -> [w300]
    shift-right: [w301] -> _
    shift-left: _ -> [w299]
    shift-right: [w297] -> _
    shift-left: 0 -> [w298]
    stop <- w303 stop-if-true
    n133 = Preview Queue Element(queue=w304, timeout in ms (-1)=w298) -> (queue out=w307:refnum<queue>, element=w308:string)  [unwired: 1 in, 2 out]
    n134 = Match Pattern(string=w308, regular expression=":") -> (before substring=w306:string, after substring=w305:string)  [unwired: 1 in, 2 out]
    n135 = case shown="\"abs\"" w306 {
      tunnel: w307 -> [_ _ _ w342 w343 w350 w355]
      tunnel: w305 -> [_ w323 w335 _ _ _ _]
      tunnel: [_ _ _ _ _ TRUE _] -> w303
      tunnel: [w316 w325 w331 w340 refnum<visa-resource-name> refnum ("VISA resource name out") w347 w352] -> w302
      tunnel: [w315 w326 w332 w339 w345 w348 w351] -> w301
      tunnel: w300 -> [w318 w328 w333 w340 w346 w347 _]
      tunnel: w299 -> [w317 w327 w334 w339 _ w348 _]
      tunnel: [_ _ _ -1 _ _ _] -> w297
      frame "idle", Default {
        n136 = local read "ESP Axis"() -> (w310:i32)
        n137 = local read "ESP_t0"() -> (w313:dbl)
        n138 = call "Read absolute position.vi"("error in (no error)"=w317, "Axis (1)"=w310, "VISA resource name"=w318) -> ("error out"=w315:errorcluster, "Position (units)"=w314:dbl, "VISA resource name out"=w316:refnum<visa-resource-name>)  [unwired: 2 in]
        "ESP_pos" <- w314
        n139 = call "mm2time.vi"("fs?"=TRUE, "Offset (mm)"=w313, "distance (mm)"=w314) -> ("time in fs/ps seconds"=→"ESP_delay":dbl)
      }
      frame "rel" {
        n140 = Match Pattern(string=w323, regular expression=":") -> (before substring=w322:string, after substring=w321:string)  [unwired: 1 in, 2 out]
        n141 = Decimal String To Number(string=w322) -> (number=w320:i32)  [unwired: 2 in, 1 out]
        n142 = Fract/Exp String To Number(string=w321) -> (number=w319:dbl)  [unwired: 3 in, 1 out]
        n143 = call "Move Relative.vi"("error in (no error)"=w327, "Position (0 units)"=w319, "Axis (1)"=w320, "VISA resource name"=w328) -> ("error out"=w326:errorcluster, "VISA resource name out"=w325:refnum<visa-resource-name>)  [unwired: 2 in]
      }
      frame "abs" {
        n144 = Match Pattern(string=w335, regular expression=":") -> (before substring=w337:string, after substring=w336:string)  [unwired: 1 in, 2 out]
        n145 = Decimal String To Number(string=w337) -> (number=w330:i32)  [unwired: 2 in, 1 out]
        n146 = Fract/Exp String To Number(string=w336) -> (number=w329:dbl)  [unwired: 3 in, 1 out]
        n147 = call "Move Absolute.vi"("error in (no error)"=w334, "Position (0 units)"=w329, "Axis (1)"=w330, "VISA resource name"=w333) -> ("error out"=w332:errorcluster, "VISA resource name out"=w331:refnum<visa-resource-name>)  [unwired: 2 in]
      }
      frame "suspend" {
        n148 = Dequeue Element(queue=w342) -> ()  [unwired: 2 in, 4 out]
      }
      frame "release" {
        n149 = Dequeue Element(queue=w343) -> ()  [unwired: 2 in, 4 out]
        n150 = call "Close.vi"("VISA resource name"=w346) -> ("error out"=w345:errorcluster)  [unwired: 10 in]
      }
      frame "close" {
        n151 = Release Queue(queue=w350) -> ()  [unwired: 2 in, 3 out]
      }
      frame "init" {
        n152 = Dequeue Element(queue=w355) -> ()  [unwired: 2 in, 4 out]
        n153 = call "Initialize.vi"("VISA resource name"="ESP301 VISA", "Serial Link (RS232)"=enum16{"RS232", "USB"}."USB") -> ("VISA resource name out"=w352:refnum<visa-resource-name>, "error out"=w351:errorcluster)  [unwired: 7 in]
      }
    }
  }
  n154 = while {
    tunnel: w10 -> [w363]
    shift-right: [w361] -> _
    shift-left: _ -> [w359]
    shift-right: [w360] -> _
    shift-left: _ -> [w358]
    shift-right: [w356] -> _
    shift-left: 0 -> [w357]
    stop <- w362 stop-if-true
    n155 = Preview Queue Element(queue=w363, timeout in ms (-1)=w357) -> (queue out=w366:refnum<queue>, element=w367:string)  [unwired: 1 in, 2 out]
    n156 = Match Pattern(string=w367, regular expression=":") -> (before substring=w365:string, after substring=w364:string)  [unwired: 1 in, 2 out]
    n157 = case shown="\"idle\", Default" w365 {
      tunnel: w366 -> [_ _ w384 w388 w397 w408]
      tunnel: w364 -> [_ _ _ _ _ _]
      tunnel: [_ _ _ _ TRUE _] -> w362
      tunnel: [w370 w372 w386 refnum<k5> refnum ("gateway_connection out") w395 w399] -> w361
      tunnel: [w369 w371 w385 w390 w394 w398] -> w360
      tunnel: w359 -> [w370 w372 w386 w392 w395 _]
      tunnel: w358 -> [w369 w371 w385 _ w394 _]
      tunnel: [_ _ -1 _ _ _] -> w356
      frame "idle", Default {
      }
      frame "relative" {
        n158 = disable-structure shown="Disabled" {
          frame Disabled {
            n159 = case shown="True" FALSE {
              tunnel: [_ w382] -> w374
              frame False {
              }
              frame True {
                n160 = call "sp_manip_get_axis_status.vi"("gateway_connection"=w382) -> ("error out"=w377:errorcluster, "axis_out"=w381:T5, "gateway_connection out"=w375:refnum<k5>)  [unwired: 6 in, 2 out]
                n161 = Index Array(array=w381) -> (element=w380:T6, index=w383:i32)
                n162 = Unbundle By Name(w380) -> ("Axis_Name"=w376:string)  [unwired: 1 out]
                n163 = Build Array(w376) -> (w379:string[])
                n164 = Build Array() -> (w378:void[])  [unwired: 1 in]
                n165 = call "sp_manip_start_move.vi"("error in"=w377, "target positions"=w378, "axis names"=w379, "gateway_connection"=w375) -> ()  [unwired: 4 in, 4 out]
              }
            }
          }
          frame Enabled {
          }
        }
      }
      frame "suspend" {
        n166 = Dequeue Element(queue=w384) -> ()  [unwired: 2 in, 4 out]
      }
      frame "release" {
        n167 = Dequeue Element(queue=w388) -> ()  [unwired: 2 in, 4 out]
        n168 = call "sp_manip_disconnect.vi"("gateway_connection"=w392) -> ("error out"=w391:errorcluster, "gateway_connection_out"=w393:refnum<k5>)  [unwired: 7 in, 2 out]
        n169 = call "tcp_gateway_close_connection.vi"("error in"=w391, "server_connection"=w393) -> ("error out"=w390:errorcluster)  [unwired: 5 in]
      }
      frame "close" {
        n170 = Release Queue(queue=w397) -> ()  [unwired: 2 in, 3 out]
      }
      frame "init" {
        n171 = Dequeue Element(queue=w408) -> ()  [unwired: 2 in, 4 out]
        n172 = call "tcp_gateway_open_connection.vi"() -> ("gateway_connection"=w403:refnum<k5>, "error out"=w402:errorcluster)  [unwired: 5 in, 3 out]
        n173 = call "sp_manip_connect.vi"("error in"=w402, "gateway_connection"=w403) -> ("error out"=w398:errorcluster, "axis_out"=w401:T5, "gateway_connection out"=w399:refnum<k5>)  [unwired: 5 in, 2 out]
        n174 = for {
          tunnel: w401 -> [w411] mode=indexing
          tunnel: [w410] -> w406 mode=indexing
          tunnel: [w409] -> w407 mode=indexing
          n175 = Unbundle By Name(w411) -> ("Axis_Name"=w410:string, "Axis_Position"=w409:dbl)
        }
        "names" <- w406
        "pos" <- w407
        n176 = control-ref of="meas_axis"() -> (w400:refnum<vi>)
        n177 = local write "dest"(w407) -> ()
        n178 = Build Array (concatenate)(w406, "XY") -> (w404:string[])
        n179 = property on="Property Node" class="CmbBox"(reference=w400, "Strings[]"=w404) -> ()  [unwired: 1 in, 2 out]
      }
    }
  }
  n180 = while {
    tunnel: w9 -> [w422]
    shift-right: [w419] -> _
    shift-left: 0 -> [w420]
    shift-right: [w418] -> _
    shift-left: _ -> [w417]
    shift-right: [w416] -> _
    shift-left: _ -> [w415]
    shift-right: [w414] -> _
    shift-left: u32 0 ("pHandle") -> [w413]
    tunnel: string[] ["Kinetic Energy", "Pass Energy", "Coil Current", "Work Function", "Detector Voltage", "Screen Voltage", "Conversion Voltage", "Focus Displacement 1", "Focus Displacement 2"] -> [w412]
    stop <- w421 stop-if-true
    n181 = Preview Queue Element(queue=w422, timeout in ms (-1)=w420) -> (queue out=w425:refnum<queue>, element=w426:string)  [unwired: 1 in, 2 out]
    n182 = Match Pattern(string=w426, regular expression=":") -> (before substring=w424:string, after substring=w423:string)  [unwired: 1 in, 2 out]
    n183 = case shown="\"idle\", Default" w424 {
      tunnel: w425 -> [_ w479 w495 w511 w525 w529 w535]
      tunnel: w423 -> [_ _ _ _ _ _ _]
      tunnel: [_ _ _ _ TRUE _ _] -> w421
      tunnel: [_ _ _ _ _ -1 _] -> w419
      tunnel: [w436 w481 w498 w509 w523 w528 w532] -> w418
      tunnel: w417 -> [w447 w470 w500 w510 w523 w528 _]
      tunnel: [w435 w480 w497 w508 w521 w526 w531] -> w416
      tunnel: w415 -> [w445 w469 w499 _ w521 w526 _]
      tunnel: [w433 w467 w496 w507 w522 w527 w534] -> w414
      tunnel: w413 -> [w433 w467 w496 w506 w522 w527 _]
      tunnel: w412 -> [w434 w460 _ _ _ _ _]
      frame "idle", Default {
        n184 = call "SL2_AD_DLL_Phoibos_GetDeviceState.vi"("dll_path"=w447, "pHandle_in"=w433, "dev_type"=DEF_dev_type."devA (analyzer)", "error in"=w445) -> ("path out"=w432:path, "state"=→"state":T1, "error out"=w431:errorcluster)  [unwired: 2 in]
        n185 = for {
          tunnel: w433 -> [w454]
          tunnel: w434 -> [w452] mode=indexing
          tunnel: [w451] -> w444 mode=indexing
          tunnel: [w450] -> w436
          shift-right: [w449] -> w435
          shift-left: w431 -> [w453]
          tunnel: w432 -> [w448]
          n186 = call "SL2_AD_DLL_Phoibos_GetVoltage.vi"("error in"=w453, "voltage_name"=w452, "pHandle"=w454, "dll path in"=w448) -> ("error out"=w449:errorcluster, "value"=w451:dbl, "dll path out"=w450:path)  [unwired: 3 in]
        }
        n187 = Index Array(array=w444) -> (element #1=→"phoib_I_1":dbl, element #2=→"phoib_I_2":dbl, element #3=→"phoib_I_3":dbl, element #4=→"phoib_I_4":dbl, element #5=→"phoib_I_5":dbl, element #6=→"phoib_I_6":dbl, element #7=→"phoib_I_7":dbl, element #8=→"phoib_I_8":dbl, element #9=→"phoib_I_9":dbl)  [unwired: 9 in]
      }
      frame "set" {
        n188 = Dequeue Element(queue=w479) -> ()  [unwired: 2 in, 4 out]
        n189 = Multiply(x="VoltageRange", y=13) -> (x*y=w476:i32)
        n190 = Add(x="Mode", y=w476) -> (x+y=w473:i32)
        n191 = Index Array(array=u32[] [251749632, 251749633, 251749634, 251749635, 251749636, 251749637, 251749638, 251749639, 251749640, 251749641, 251749642, 251749643, 251749644, 251749645, 251749646, 251749647, 251749648, 251749649, 251749650, 251749651, 251749652, 251749653, 251749654, 251749655, 251749656, 251749657, 251749658, 251749659, 251749660, 251749661, 251749662, 251749663, 251749664, 251749665, 251749666, 251749667, 251749668, 251749669, 251749670, 251749671, 251749672, 251749673, 251749674, 251749675, 251749676, 251749677, 251749678, 251749679, 251749680, 251749681, 251749682, 251749683, 251749684, 251749685, 251749686, 251749687, 251749688, 251749689, 251749690, 251749691, 251749692, 251749693, 251749694, 251749695, 251749696] ("modeIDs"), index=w473) -> (element=w471:u32)
        n192 = Build Array("phoib_I_1s", "phoib_I_2s", "phoib_I_3s", "phoib_I_4s", "phoib_I_5s", "phoib_I_6s", "phoib_I_7s", "phoib_I_8s", "phoib_I_9s") -> (w459:dbl[])
        n193 = call "SL2_AD_DLL_Phoibos_SetDeviceMode.vi"("pHandle"=w467, "error in"=w469, "value"=w471, "dev_type"=DEF_dev_type."devA (analyzer)", "dll path in"=w470) -> ("error out"=w458:errorcluster, "dll path out"=w468:path)  [unwired: 4 in]
        n194 = for {
          tunnel: w467 -> [w487]
          shift-right: [w494] -> w481
          shift-left: w468 -> [w491]
          tunnel: w460 -> [w486] mode=indexing
          tunnel: w459 -> [w485] mode=indexing
          shift-right: [w493] -> w480
          shift-left: w458 -> [w489]
          n195 = call "SL2_AD_DLL_Phoibos_GetVoltageRange.vi"("error in"=w489, "voltage_name"=w486, "pHandle"=w487, "dll path in"=w491) -> ("error out"=w488:errorcluster, "min"=w483:dbl, "max"=w484:dbl, "dll path out"=w490:path)  [unwired: 2 in]
          n196 = In Range and Coerce(upper limit=w484, x=w485, lower limit=w483) -> (coerced(x)=w482:dbl)  [unwired: 1 out]
          n197 = call "SL2_AD_DLL_Phoibos_SetVoltage.vi"("commit"=TRUE, "pHandle"=w487, "error in"=w488, "value"=w482, "voltageName"=w486, "dll path in"=w490) -> ("error out"=w493:errorcluster, "dll path out"=w494:path)  [unwired: 3 in]
        }
      }
      frame "standby" {
        w501 = T1 0 items=["Off"=-1, "Standby"=0, "On"=1] ("state")
        n198 = Dequeue Element(queue=w495) -> ()  [unwired: 2 in, 4 out]
        n199 = call "SL2_AD_DLL_Phoibos_SetDeviceState.vi"("pHandle_in"=w496, "error in"=w499, "state"=w501, "dev_type"=DEF_dev_type."devA (analyzer)", "dll_path"=w500) -> ("error out"=w497:errorcluster, "path out"=w498:path)  [unwired: 2 in]
      }
      frame "release" {
        n200 = Dequeue Element(queue=w511) -> ()  [unwired: 2 in, 4 out]
        n201 = flat-sequence {
          tunnel: w510 -> [w512]
          tunnel: w506 -> [w513]
          tunnel: [w516] -> w505
          tunnel: [w515] -> w504
          tunnel: [u32 0] -> w503
          tunnel: [w518] -> w507
          tunnel: [w519] -> w508
          tunnel: [w520] -> w509
          tunnel: w505 -> [w520]
          tunnel: w504 -> [w519]
          tunnel: w503 -> [w518]
          frame #0 {
            n202 = call "SL2_AD_DLL_Phoibos_Shutdown.vi"("pHandle"=w513, "dll path in"=w512) -> ("error out"=w515:errorcluster, "dll path out"=w516:path)  [unwired: 4 in]
          }
          frame #1 {
            n203 = local write "phoib_con?"(FALSE ("phoib_con?")) -> ()
          }
        }
      }
      frame "close" {
        n204 = Release Queue(queue=w525) -> ()  [unwired: 2 in, 3 out]
      }
      frame "suspend" {
        n205 = Dequeue Element(queue=w529) -> ()  [unwired: 2 in, 4 out]
      }
      frame "init" {
        n206 = Dequeue Element(queue=w535) -> ()  [unwired: 2 in, 4 out]
        n207 = flat-sequence {
          tunnel: [w542] -> w533
          tunnel: [w538] -> w532
          tunnel: [w537] -> w531
          tunnel: [w550] -> w534
          tunnel: w533 -> [w550]
          frame #0 {
            n208 = local write "phoib_con?"(FALSE ("phoib_con?")) -> ()
          }
          frame #1 {
            w541 = DEF_dev_type."devA (analyzer)" ("dev_type")
            n209 = call "GetSL2AD_VI_dllPath.vi"() -> ("error"=w545:errorcluster, "Path"=w546:path)  [unwired: 9 in, 1 out]
            n210 = call "SL2_AD_DLL_List_Devices.vi"("error in"=w545, "dev_type"=w541, "dll path in"=w546) -> ("error out"=w539:errorcluster, "devices"=w548:string[], "dll path out"=w540:path)  [unwired: 2 in]
            n211 = Index Array(array=w548) -> (element=w547:string)  [unwired: 1 in]
            n212 = call "SL2_AD_DLL_Phoibos_Initialize.vi"("error in"=w539, "analyzerId"=w547, "dll_path"=w540) -> ("error out"=w543:errorcluster, "pHandle"=w542:u32, "path out"=w544:path)  [unwired: 2 in]
            n213 = call "SL2_AD_DLL_Phoibos_ListDeviceModes.vi"("dll path in"=w544, "dev_type"=w541, "pHandle"=w542, "error in"=w543) -> ("dll path out"=w538:path, "error out"=w537:errorcluster)  [unwired: 1 in, 2 out]
          }
          frame #2 {
            n214 = local write "phoib_con?"(TRUE ("phoib_con?")) -> ()
          }
        }
      }
    }
    "error out 2" <- w416
  }
